vi "VibSerialCheck.vi"(11 "VISA Refnum in":refnum<visa-resource-name>) -> (0 "NoSerial":refnum<visa-resource-name>="No Serial", 3 "Serial?":bool)   [LabVIEW 2022 SP3]
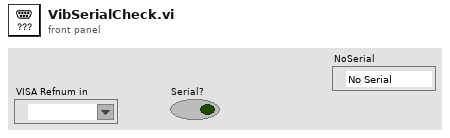
[diagram p1: front panel]
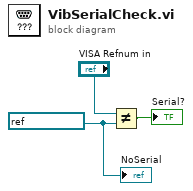
[diagram p0: block diagram]
diagram:
  w1 = refnum<visa-resource-name> "No Serial" ("y")
  n1 = Not Equal?(x="VISA Refnum in", y=w1) -> (x != y?=→"Serial?":bool)
  "NoSerial" <- w1
